vi "Configure Multi Eval Meas Spectrum SEM.vi"(7 "SEM Statistic Count (20)":i32=20, 8 "error in (no error)":errorcluster, 9 "SEM Enabled (Off)":bool, 10 "Instance (1)":T1=1, 11 "VISA resource name":refnum<visa-resource-name>) -> (0 "error out":errorcluster, 3 "VISA resource name out":refnum<visa-resource-name>)   [LabVIEW 2020, in "Rohde&Schwarz CMXP NR FR2 Measurement.lvlib"]
doc: "Enables and configures the evaluation of SEM results in the multi-evaluation measurement.\n\nAttributes:\nRSCMXPNRFR2M_ATTR_MULTI_EVAL_MEASUREMENT_SPECTRUM_SEM_ENABLED\nRSCMXPNRFR2M_ATTR_MULTI_EVAL_MEASUREMENT_SPECTRUM_SEM_STATISTIC_COUNT\n\nRemote-control commands:\nCONFigure:NRMMw:MEAS<i>:MEValuation:RESult:SEMask\nCONFigure:NRMMw:MEAS<i>:MEValuation:SCOunt:SPECtrum:SEMask"
uses:
  <instrlib>/Rohde&Schwarz CMXP NR FR2 Measurement/Rohde&Schwarz CMXP NR FR2 Measurement.lvlib
  <instrlib>/Rohde&Schwarz CMXP NR FR2 Measurement/Private/_Instance.ctl
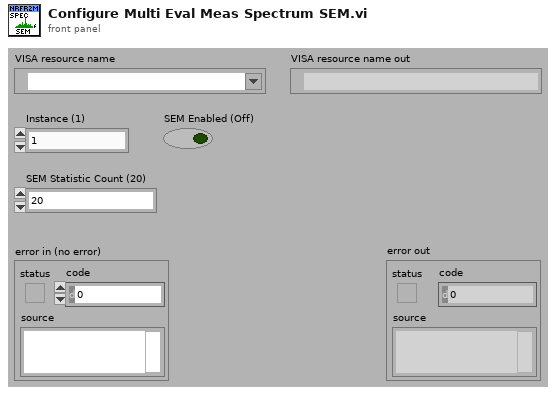
[diagram p1: front panel]
types:
  T1 = typedef "Rohde&Schwarz CMXP NR FR2 Measurement.lvlib/_Instance.ctl" = i32
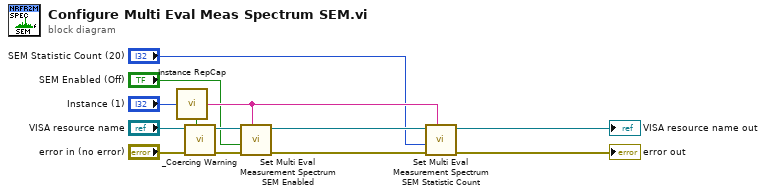
[diagram p0: block diagram]
diagram:
  n1 = call <instrlib>:"Instance RepCap.vi"("Instance In"="Instance (1)") -> ("In Range?"=w11:bool, "RepCap Identifier Out"=w8:string)  [unwired: 1 in]
  n2 = call <instrlib>:"_Coercing Warning.vi"("In Range?"=w11, "error in (no error)"="error in (no error)", "VISA resource name"="VISA resource name") -> ("error out"=w9:errorcluster, "VISA resource name out"=w10:refnum<visa-resource-name>)  [unwired: 7 in]
  n3 = call "Set Multi Eval Measurement Spectrum SEM Enabled"("Repeated Capabilities"=w8, "error in (no error)"=w9, "Multi Eval Measurement Spectrum SEM Enabled (OFF)"="SEM Enabled (Off)", "instrument handle"=w10) -> ("error out"=w7:errorcluster, "instrument handle out"=w6:refnum<visa-resource-name>)  [unwired: 6 in]
  n4 = call "Set Multi Eval Measurement Spectrum SEM Statistic Count"("Repeated Capabilities"=w8, "error in (no error)"=w7, "Multi Eval Measurement Spectrum SEM Statistic Count (0)"="SEM Statistic Count (20)", "instrument handle"=w6) -> ("error out"=→"error out":errorcluster, "instrument handle out"=→"VISA resource name out":refnum<visa-resource-name>)  [unwired: 6 in]
